vi "2D Feather Plot.vi"() -> ()   [LabVIEW 2017, in "2D_Merge.lvlib"]
uses:
  <vilib>/Math Plots/2D Math Plots/Merge VIs/2D_Merge.lvlib
  <vilib>/Math Plots/2D Math Plots/2D Feather/2D Feather XCtrl/2D Feather.xctl
  <vilib>/Math Plots/2D Math Plots/2D Feather/2D Feather Datatype/Public/Plot Helper (Vector).vi
  <vilib>/Math Plots/2D Math Plots/2D Feather/2D Feather Datatype/2D Feather Datatype.lvclass
panel:
  out "2D Feather":refnum<class "2D Plot Datatype.lvclass">[](xcontrol)
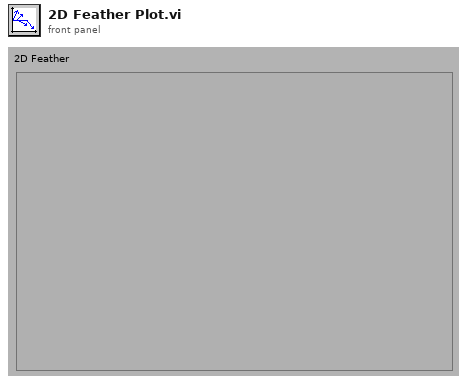
[diagram p1: front panel]
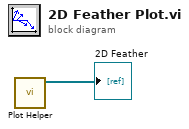
[diagram p0: block diagram]
diagram:
  n1 = call-poly <vilib>:"Plot Helper.vi"() -> ("2D Plot Class Obj Array out"=→"2D Feather":refnum<class "2D Plot Datatype.lvclass">[])  [unwired: 4 in, 7 out]
